vi "Save.vi"(8 "error in":errorcluster, 11 "SpreadsheetDocument in":refnum<k24>) -> (0 "error out":errorcluster, 3 "SpreadsheetDocument out":refnum<k24>)   [LabVIEW 2021, in "Open Xml.lvlib"]
uses:
  Open Xml.lvlib
  D:/git/Open-Xml-LabVIEW/dll/DocumentFormat.OpenXml.dll
  dll/DocumentFormat.OpenXml.dll
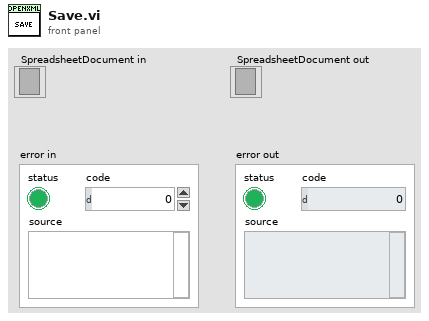
[diagram p1: front panel]
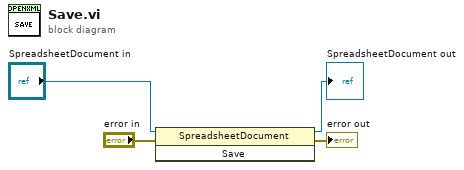
[diagram p0: block diagram]
diagram:
  n1 = invoke class="SpreadsheetDocument" method="Save"(reference="SpreadsheetDocument in", error in="error in") -> (reference out=→"SpreadsheetDocument out":refnum<k24>, error out=→"error out":errorcluster)  [unwired: 1 in, 1 out]
